vi "testMaxFileSize (database - not exceeded).vi"(8 "error in (no error)":errorcluster, 11 "TestCase in":refnum<class "Test Max File Size (SQL).lvclass">) -> (0 "error out":errorcluster, 3 "TestCase out":refnum<class "Test Max File Size (SQL).lvclass">)   [LabVIEW 2019, in "Test Max File Size (SQL).lvclass"]
uses:
  Test Max File Size (SQL).lvclass
  Test Max File Size (SQL).lvclass/Test Max File Size (SQL).ctl
  Program Files (x86)/National Instruments/LabVIEW 2019/vi.lib/addons/_TSC/TSC Event Logger/Log/Event Level.ctl
  Program Files (x86)/National Instruments/LabVIEW 2019/vi.lib/addons/_TSC/TSC Event Logger/TSC Event Logger.lvlib
  Program Files (x86)/National Instruments/LabVIEW 2019/vi.lib/addons/_TSC/TSC Event Logger/Log/Log.lvclass
  9400858f-8242-4f0f-a3a8-0c5d1ac263e7.vi
  Log Sinks/SQLite Database/SQLite Database.lvclass
  1899192f-cf69-4381-8047-4ca8678618ad.vi
  Program Files (x86)/National Instruments/LabVIEW 2019/vi.lib/addons/_TSC/TSC Event Logger/Log Sinks/Log Sinks.lvclass
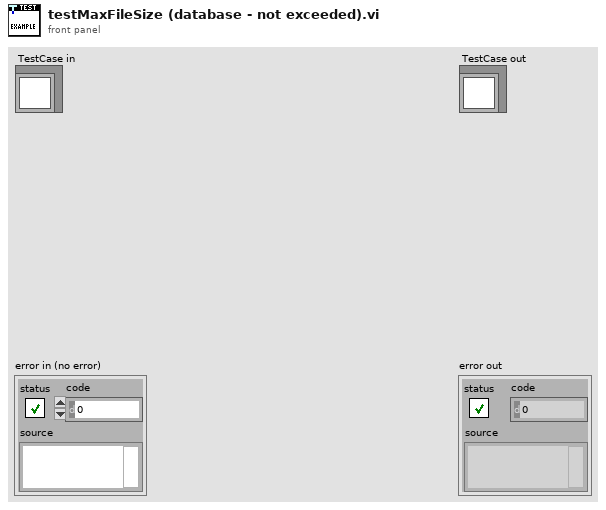
[diagram p1: front panel]
types:
  T1 = typedef "TSC Event Logger.lvlib/Event Level.ctl" = enum16{"OFF", "TRACE", "DEBUG", "INFO", "WARN", "ERROR", "FATAL"}
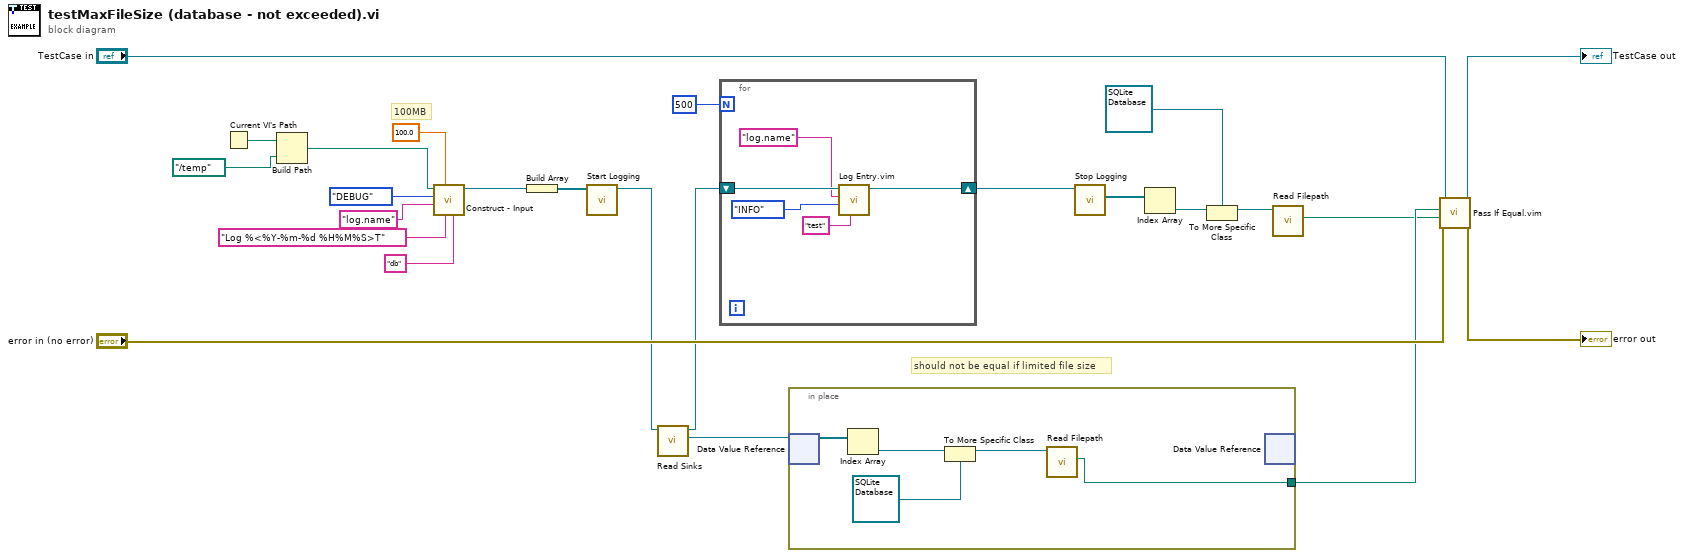
[diagram p0: block diagram]
diagram:
  # "100MB"
  # "should not be equal if limited file size"
  n1 = Current VI's Path() -> (path=w10:path)
  n2 = Build Path(base path=w10, name or relative path=path "../temp") -> (appended path=w12:path)
  n3 = call "Construct - Input.vi"("extension"="db", "file name format"="Log %<%Y-%m-%d %H%M%S>T", "Max File Size (MB)"=100.0, "Name"="log.name", "Level"=Event_Level."DEBUG", "log location"=w12) -> ("SQLite Database out"=w5:refnum<class "SQLite Database.lvclass">)  [unwired: 4 in, 1 out]
  n4 = Build Array(w5) -> (w4:refnum<class "SQLite Database.lvclass">[])
  n5 = call "Start Logging.vi"("Sinks"=w4) -> ("Logger"=w2:refnum<class "Log.lvclass">)  [unwired: 9 in, 1 out]
  n6 = call "Read Sinks.vi"("Log in"=w2) -> ("Sink DVR Array"=w21:refnum<data-value>, "Log out"=w16:refnum<class "Log.lvclass">)  [unwired: 9 in]
  n7 = for {
    N: 500 -> [_]
    shift-right: [w28] -> w17
    shift-left: w16 -> [w29]
    n8 = call "Log Entry.vim"("Message"="test", "Level"=Event_Level."INFO", "Logger"="log.name", "Log in"=w29) -> ("Log out"=w28:refnum<class "Log.lvclass">)  [unwired: 6 in, 1 out]
  }
  n9 = in-place {
    in-place-border: [w31] -> w20
    n10 = in-place-dvr #1(w21) -> (w35:refnum<class "Log Sinks.lvclass">[])  [unwired: 1 out]
    n11 = Index Array(array=w35) -> (element=w34:refnum<class "Log Sinks.lvclass">)  [unwired: 1 in]
    n12 = To More Specific Class(target class=refnum<class "SQLite Database.lvclass"> refnum ("TSC Event Logger.lvlib:SQLite Database.lvclass"), reference=w34) -> (specific class reference=w33:refnum<class "SQLite Database.lvclass">)  [unwired: 1 in, 1 out]
    n13 = call "Read Filepath.vi"("SQLite Database in"=w33) -> ("File Path Indicator"=w31:path)  [unwired: 9 in, 1 out]
    n14 = in-place-dvr #1() -> ()  [unwired: 1 in, 2 out]
  }
  n15 = call "Stop Logging.vi"("Logger"=w17) -> ("sinks"=w13:refnum<class "Log Sinks.lvclass">[])  [unwired: 9 in, 1 out]
  n16 = Index Array(array=w13) -> (element=w15:refnum<class "Log Sinks.lvclass">)  [unwired: 1 in]
  n17 = To More Specific Class(target class=refnum<class "SQLite Database.lvclass"> refnum ("TSC Event Logger.lvlib:SQLite Database.lvclass"), reference=w15) -> (specific class reference=w14:refnum<class "SQLite Database.lvclass">)  [unwired: 1 in, 1 out]
  n18 = call "Read Filepath.vi"("SQLite Database in"=w14) -> ("File Path Indicator"=w18:path)  [unwired: 9 in, 1 out]
  n19 = call "Pass If Equal.vim"("error in (no error)"="error in (no error)", "Actual"=w18, "Expected"=w20, "LUnit Test Case In"="TestCase in") -> ("error out"=→"error out":errorcluster, "LUnit Test Case Out"=→"TestCase out":refnum<class "Test Max File Size (SQL).lvclass">)  [unwired: 6 in]
